vi "TDMS Copy Channel.vi"(5 "channel name":string, 7 "group name":string, 8 "error in":errorcluster, 10 "tdms dest in":refnum<k34>, 11 "tdms source in":refnum<k34>) -> (0 "error out":errorcluster, 2 "tdms dest out":refnum<k34>, 3 "tdms source out":refnum<k34>)   [LabVIEW 2011]
doc: "Copies the properties and the data in Channel from the source file to the destination file. Existing properties become overwritten and the new data is appended to the old one if present."
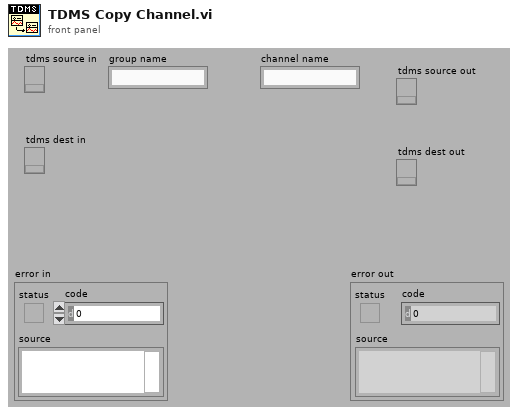
[diagram p1: front panel]
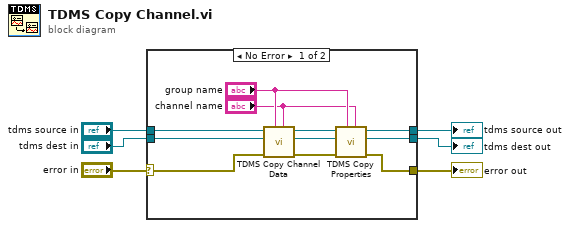
[diagram p0: block diagram]
diagram:
  n1 = case shown="No Error" "error in" {
    selector: "error in" -> [w7 w20]
    tunnel: [w17 w19] -> w6
    tunnel: [w16 w18] -> w5
    tunnel: "tdms source in" -> [w15 w19]
    tunnel: "tdms dest in" -> [w13 w18]
    tunnel: [w8 w20] -> w2
    frame No Error {
      n2 = call "TDMS Copy Channel Data.vi"("channel name"="channel name", "group name"="group name", "error in"=w7, "tdms dest in"=w13, "tdms source in"=w15) -> ("error out"=w14:errorcluster, "tdms dest out"=w12:refnum<k34>, "tdms source out"=w11:refnum<k34>)  [unwired: 4 out]
      n3 = call "TDMS Copy Properties.vi"("channel name"="channel name", "group name"="group name", "error in"=w14, "tdms dest in"=w12, "tdms source in"=w11) -> ("error out"=w8:errorcluster, "tdms dest out"=w16:refnum<k34>, "tdms source out"=w17:refnum<k34>)  [unwired: 4 out]
    }
    frame Error {
    }
  }
  "tdms source out" <- w6
  "tdms dest out" <- w5
  "error out" <- w2
